vi "View.vi"(0 "object in":refnum<class "Client.lvclass">, 5 "error in (no error)":errorcluster) -> (14 "object out":refnum<class "Client.lvclass">, 16 "Message":T1, 19 "error out":errorcluster)   [LabVIEW 2024, in "Client.lvclass"]
doc: "Read the file and return data"
uses:
  Client.lvclass
  Support/Type Def/Message.ctl
  Client.lvclass/Client.ctl
  Support/Type Def/Requirements.ctl
  Support/Type Def/File Type.ctl
  Support/Type Def/Data.ctl
  Abstractions/DataType/DataType.lvclass
panel:
  # "Connector Pane"
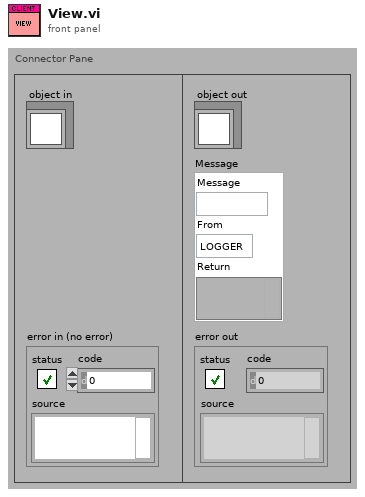
[diagram p1: front panel]
types:
  T1 = typedef "Message.ctl" = cluster{"Message":string, "From":enum16{"LOGGER", "VIEWER"}, "Return":variant}
  T2 = typedef "Data.ctl" = map{string, dbl[]}
  T3 = typedef "Requirements.ctl" = cluster{"From":T4, "File Handler":variant, "Input":variant}
  T4 = typedef "File Type.ctl" = enum32{"TDMS", "EXCEL"}
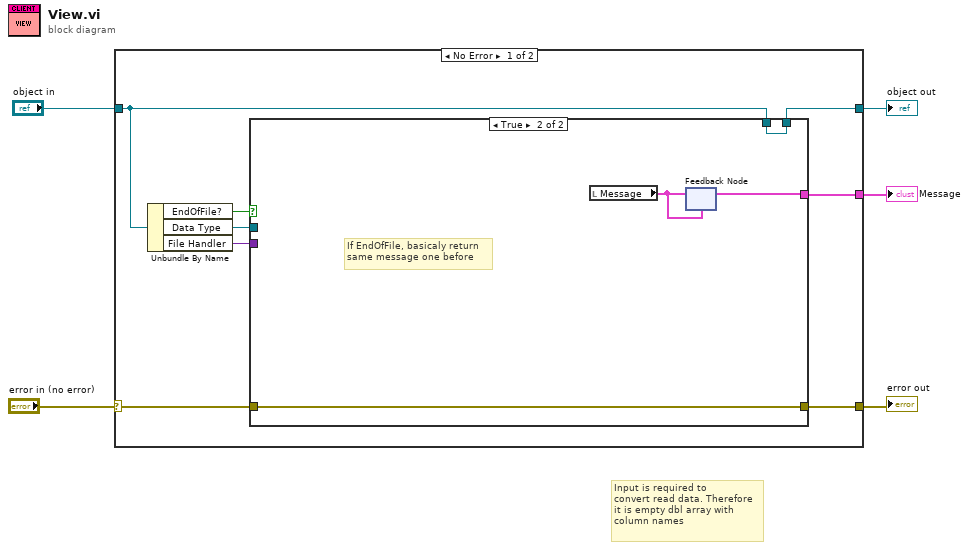
[diagram p0: block diagram]
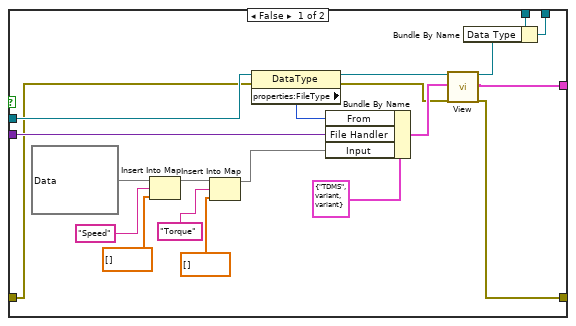
[diagram p2: hidden frame]
diagram:
  # "Input is required to\nconvert read data. Therefore\nit is empty dbl array with\ncolumn names"
  n1 = case shown="No Error" "error in (no error)" {
    selector: "error in (no error)" -> [w7 w39]
    tunnel: [w6 w39] -> w4
    tunnel: [w10 w38] -> w2
    tunnel: "object in" -> [w9 w38]
    tunnel: [w8 _] -> w1
    frame No Error {
      n2 = Unbundle By Name(w9) -> ("EndOfFile?"=w11:bool, "Data Type"=w13:refnum<class "DataType.lvclass">, "File Handler"=w12:variant)
      n3 = case shown="True" w11 {
        tunnel: w13 -> [w33 _]
        tunnel: w12 -> [w29 _]
        tunnel: w9 -> [w20 w35]
        tunnel: [w19 w35] -> w10
        tunnel: [w16 w37] -> w8
        tunnel: w7 -> [w15 w34]
        tunnel: [w14 w34] -> w6
        frame False {
          n4 = Insert Into Map(map in=T2 {} ("Data"), key="Speed", value=dbl[] []) -> (map out=w26:T2)  [unwired: 2 out]
          n5 = Insert Into Map(map in=w26, key="Torque", value=dbl[] []) -> (map out=w21:T2)  [unwired: 2 out]
          n6 = property class="DataType"(reference=w33, error in=w15) -> (reference out=w31:refnum<class "DataType.lvclass">, error out=w17:errorcluster, "properties:FileType"=w30:T4)
          n7 = Bundle By Name(cluster=T3 {"From"=enum."TDMS", "File Handler"=variant, "Input"=variant} ("Requirements"), "From"=w30, "File Handler"=w29, "Input"=w21) -> (w28:T3)
          n8 = call-dynamic "View.vi"("object in"=w31, "Requirements"=w28, "error in (no error)"=w17) -> ("object out"=w18:refnum<class "DataType.lvclass">, "Message"=w16:T1, "error out"=w14:errorcluster)  [unwired: 14 in]
          n9 = Bundle By Name(cluster=w20, "Data Type"=w18) -> (w19:refnum<class "Client.lvclass">)
        }
        frame True {
          # "If EndOfFile, basicaly return\nsame message one before"
          n10 = local read "Message"() -> (w36:T1)
          n11 = feedback-in #1(w36) -> ()
          n12 = feedback #1(w36) -> (w37:T1)
        }
      }
    }
    frame Error {
    }
  }
  "error out" <- w4
  "object out" <- w2
  "Message" <- w1
